vi "Car Position Moved.vi"(8 "error in (no error)":errorcluster, 10 "Vehicle Position":T1, 11 "Car Wash Controller in":refnum<class "Car Wash Controller.lvclass">) -> (0 "error out":errorcluster, 3 "Car Wash Controller out":refnum<class "Car Wash Controller.lvclass">)   [LabVIEW 2012, in "Car Wash Controller.lvlib" / "Car Wash Controller.lvclass"]
uses:
  Car Wash Controller.lvclass
  Car Wash Controller State.ctl
  Vehicle Position.ctl
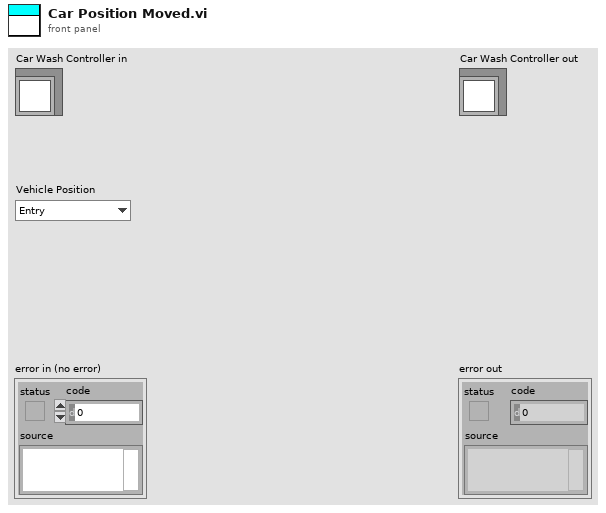
[diagram p1: front panel]
types:
  T1 = typedef "Car Wash Controller.lvlib/Car Wash Controller.lvclass/Vehicle Position.ctl" = enum16{"Entry", "Station 1", "Station 2", "Station 3", "Exit"}
  T2 = typedef "Car Wash Controller.lvlib/Car Wash Controller.lvclass/Car Wash Controller State.ctl" = enum16{"Initial State", "Wait For Start State", "Start State", "Wait For Vehicle Position State", "Wash Step Execution State", "Wash Step / Cycle Completion State", "Wash Exit State", "Wash Abort / Terminate State"}
  T3 = typedef "Car Wash Controller.lvlib/Car Wash Controller.lvclass/Wash Step.ctl" = enum16{"Under Body Wash", "Bug Remover", "Pre-Soak", "High Pressure Wash", "Low Pressure Wax", "Spot Free Rince", "Tire Shine Foam", "Air Dry"}
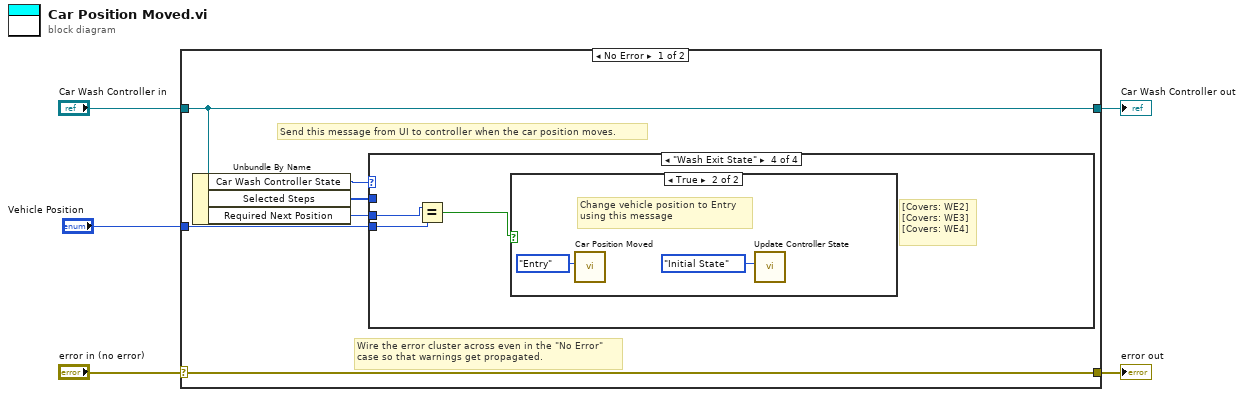
[diagram p0: block diagram]
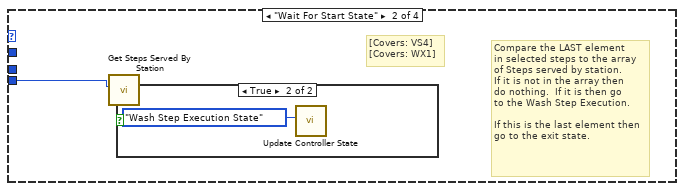
[diagram p3: hidden frame]
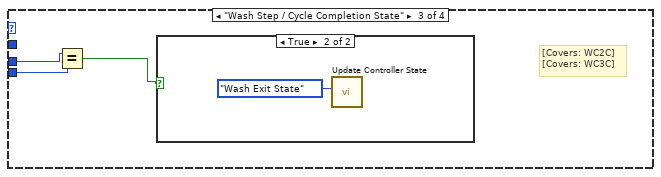
[diagram p5: hidden frame]
diagram:
  n1 = case shown="No Error" "error in (no error)" {
    selector: "error in (no error)" -> [w11 w24]
    tunnel: [w11 w24] -> w4
    tunnel: [w10 w23] -> w2
    tunnel: "Car Wash Controller in" -> [w10 w23]
    tunnel: "Vehicle Position" -> [w8 _]
    frame No Error {
      # "Send this message from UI to controller when the car position moves."
      # "Wire the error cluster across even in the \"No Error\"\ncase so that warnings get propagated."
      n2 = Unbundle By Name(w10) -> ("Car Wash Controller State"=w9:T2, "Selected Steps"=w7:T3[], "Required Next Position"=w6:T1)
      n3 = case shown="\"Wash Exit State\"" w9 {
        tunnel: w8 -> [_ w12 w15 w19]
        tunnel: w7 -> [_ _ _ _]
        tunnel: w6 -> [_ _ w16 w20]
        frame "Initial State", Default {
        }
        frame "Wait For Start State" {
          # "[Covers: VS4]\n[Covers: WX1]"
          # "Compare the LAST element\nin selected steps to the array\nof Steps served by station.\nIf it is not in the array then\ndo nothing.  If it is then go\nto the Wash Step Execution.\n\nIf this is the last element then\ngo to the exit state."
          n4 = call "Get Steps Served By Station.vi"("Vehicle Position"=w12) -> ()  [unwired: 8 in, 3 out]
          n5 = case shown="True" {
            selector: _ -> [_ _]
            frame False {
            }
            frame True {
              n6 = call "Update Controller State.vi"("Car Wash Controller State"=Car_Wash_Controller_State."Wash Step Execution State") -> ()  [unwired: 9 in, 2 out]
            }
          }
        }
        frame "Wash Step / Cycle Completion State" {
          # "[Covers: WC2C]\n[Covers: WC3C]"
          n7 = Equal?(x=w16, y=w15) -> (x = y?=w14:bool)
          n8 = case shown="True" w14 {
            frame False {
            }
            frame True {
              n9 = call "Update Controller State.vi"("Car Wash Controller State"=Car_Wash_Controller_State."Wash Exit State") -> ()  [unwired: 9 in, 2 out]
            }
          }
        }
        frame "Wash Exit State" {
          # "[Covers: WE2]\n[Covers: WE3]\n[Covers: WE4]"
          n10 = Equal?(x=w20, y=w19) -> (x = y?=w18:bool)
          n11 = case shown="True" w18 {
            frame False {
            }
            frame True {
              # "Change vehicle position to Entry\nusing this message"
              n12 = call "Car Position Moved.vi"("Vehicle Position"=Vehicle_Position."Entry") -> ()  [unwired: 9 in, 2 out]
              n13 = call "Update Controller State.vi"("Car Wash Controller State"=Car_Wash_Controller_State."Initial State") -> ()  [unwired: 9 in, 2 out]
            }
          }
        }
      }
    }
    frame Error {
    }
  }
  "error out" <- w4
  "Car Wash Controller out" <- w2
